vi "Histogram Bin Size Dialog.vi"(8 "error in (no error)":errorcluster, 11 "Current Bin Size":dbl=nan format="%#g") -> (0 "error out":errorcluster, 1 "OK":bool, 2 "Rescale Plot_":bool, 3 "Bin Size_":dbl caption="Bin Size" format="%#g", 5 "Binning Factor_":dbl format="%#g")   [LabVIEW 2021, in "Histogram Window.lvlib"]
doc: "Displays a standard dialog box that prompts users to enter information, such as a user name and password.\n--------------------\n\nThis Express VI is configured as follows:\n\nMessage to Display to the User:Enter new histogram bin size:\nThe inputs are: \nNumber: Bin Size"
uses:
  Histogram Window.lvlib
panel:
  out "Warning":string="< 1 not supported"
  in  "Binning Factor":dbl=1.0 caption="Bin Size" min=1.0 format="%#g"
  in  "Rescale Plot":bool
  out "Current Bin Size":dbl caption="Bin Size" format="%#g"
  in  "New Bin Size":dbl caption="Bin Size" min=0.0 format="%#g"
  out "String":string="Enter new histogram bin size:"
  in  "Cancel":bool
  in  "OK":bool caption="OK2"
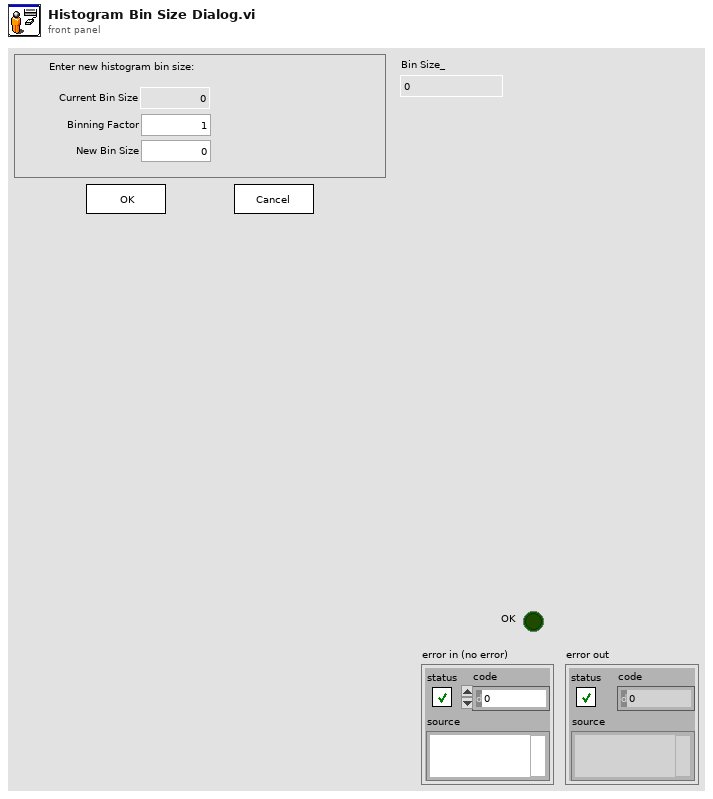
[diagram p1: front panel]
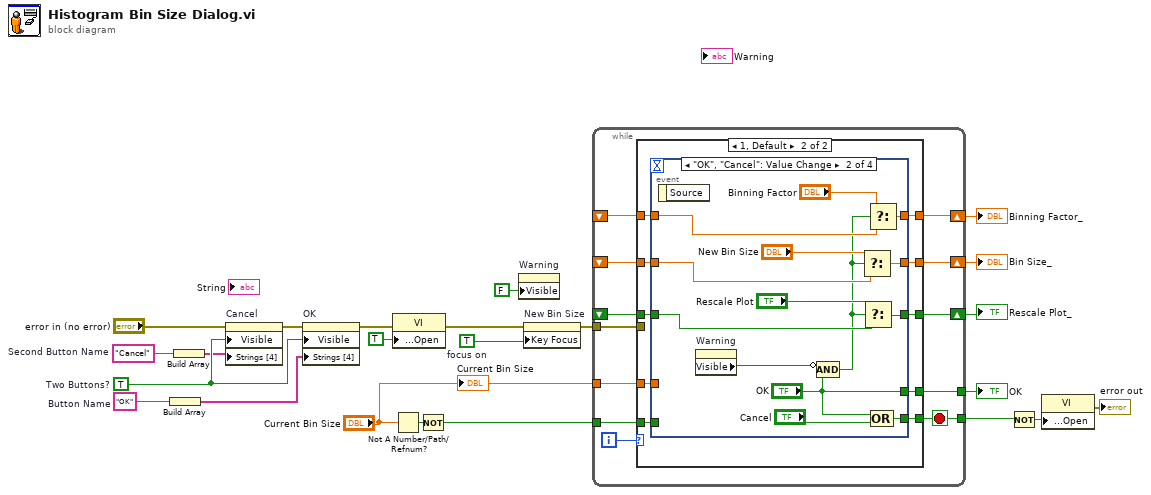
[diagram p0: block diagram]
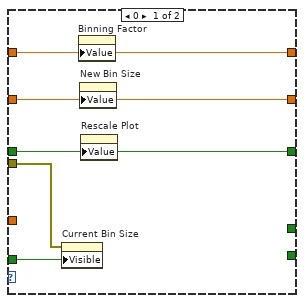
[diagram p2: hidden frame]
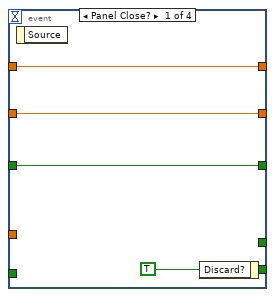
[diagram p3: hidden frame]
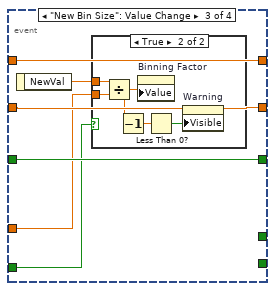
[diagram p4: hidden frame]
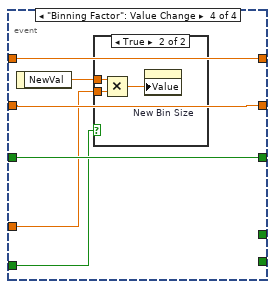
[diagram p6: hidden frame]
diagram:
  w12 = TRUE  # focus on
  w19 = "Cancel"  # Second Button Name
  w17 = "OK"  # Button Name
  w23 = TRUE  # Two Buttons?
  n1 = Build Array(w17) -> (w18:string[])
  n2 = Build Array(w19) -> (w20:string[])
  n3 = property on="Cancel" class="Bool"(error in="error in (no error)", "Visible"=w23, "Strings [4]"=w20) -> (error out=w22:errorcluster)  [unwired: 1 in, 1 out]
  n4 = property on="OK" class="Bool"(error in=w22, "Visible"=w23, "Strings [4]"=w18) -> (error out=w3:errorcluster)  [unwired: 1 in, 1 out]
  n5 = property class="VI"(error in=w3, "Front Panel Window:Open"=TRUE) -> (error out=w16:errorcluster)  [unwired: 1 in, 1 out]
  n6 = Not A Number/Path/Refnum?(number/path/refnum="Current Bin Size") -> (NaN/Path/Refnum?=w2:bool)
  n7 = Not(x=w2) -> (.not. x?=w4:bool)
  n8 = property on="Warning" class="Str"("Visible"=FALSE) -> ()  [unwired: 2 in, 2 out]
  n9 = property on="New Bin Size" class="DigNum (strict)"(error in=w16, "Key Focus"=w12) -> (error out=w5:errorcluster)  [unwired: 1 in, 1 out]
  n10 = while {
    shift-right: [w34] -> w9
    shift-left: _ -> [w33]
    shift-right: [w31] -> w10
    shift-left: _ -> [w32]
    shift-right: [w29] -> w8
    shift-left: _ -> [w30]
    tunnel: [w28] -> w11
    tunnel: [w27] -> w7
    tunnel: "Current Bin Size" -> [w26]
    tunnel: w5 -> [w25]
    tunnel: w4 -> [w24]
    i -> [w35]
    stop <- w27 stop-if-true
    n11 = case shown="1, Default" w35 {
      tunnel: [_ w50] -> w27
      tunnel: [w40 w48] -> w34
      tunnel: w33 -> [w40 w47]
      tunnel: w32 -> [w39 w45]
      tunnel: [w39 w46] -> w31
      tunnel: w30 -> [w38 w43]
      tunnel: [w38 w44] -> w29
      tunnel: [_ w49] -> w28
      tunnel: w26 -> [_ w42]
      tunnel: w25 -> [w37 _]
      tunnel: w24 -> [w36 w41]
      frame 0 {
        n12 = property on="Current Bin Size" class="DigNum (strict)"(error in=w37, "Visible"=w36) -> ()  [unwired: 1 in, 2 out]
        n13 = property on="Binning Factor" class="DigNum (strict)"("Value"=w40) -> ()  [unwired: 2 in, 2 out]
        n14 = property on="New Bin Size" class="DigNum (strict)"("Value"=w39) -> ()  [unwired: 2 in, 2 out]
        n15 = property on="Rescale Plot" class="Bool (strict)"("Value"=w38) -> ()  [unwired: 2 in, 2 out]
      }
      frame 1, Default {
        n16 = event shown="[1] \"OK\", \"Cancel\": Value Change" {
          selector: _ -> [_ _ _ _]
          dyn-events: _ -> [_ _ _ _]
          timeout: _ -> [_ _ _ _]
          tunnel: [w54 w58 _ _] -> w50
          tunnel: [_ "OK" _ _] -> w49
          tunnel: [w53 w67 w74 w85] -> w48
          tunnel: w47 -> [w53 w66 w74 w85]
          tunnel: [w52 w64 w71 w82] -> w46
          tunnel: w45 -> [w52 w63 w71 w82]
          tunnel: [w51 w61 w73 w84] -> w44
          tunnel: w43 -> [w51 w60 w73 w84]
          tunnel: w42 -> [_ _ w70 w81]
          tunnel: w41 -> [_ _ w69 w80]
          event Panel Close? {
            w54 = TRUE ("Discard?")
            n17 = event-data() -> ()  [unwired: 1 in, 1 out]
            n18 = event-data("Discard?"=w54) -> ()  [unwired: 1 in, 1 out]
          }
          event "OK", "Cancel": Value Change {
            n19 = event-data() -> ()  [unwired: 1 in, 1 out]
            n20 = property on="Warning" class="Str"() -> ("Visible"=w57:bool)  [unwired: 2 in, 2 out]
            n21 = Compound Arithmetic op=AND(invert w57, "OK") -> (w55:bool)
            n22 = Select(t="New Bin Size", s=w55, f=w63) -> (s? t:f=w64:dbl)
            n23 = Select(t="Rescale Plot", s=w55, f=w60) -> (s? t:f=w61:bool)
            n24 = Select(t="Binning Factor", s=w55, f=w66) -> (s? t:f=w67:dbl)
            n25 = Compound Arithmetic op=OR("OK", "Cancel") -> (w58:bool)
          }
          event "New Bin Size": Value Change {
            n26 = event-data() -> ("NewVal"=w72:dbl)  [unwired: 1 in]
            n27 = case shown="True" w69 {
              tunnel: w72 -> [_ w79]
              tunnel: w70 -> [_ w78]
              frame False {
              }
              frame True {
                n28 = Divide(x=w79, y=w78) -> (x/y=w77:dbl)
                n29 = Decrement(x=w77) -> (x-1=w76:dbl)
                n30 = property on="Binning Factor" class="DigNum (strict)"("Value"=w77) -> ()  [unwired: 2 in, 2 out]
                n31 = Less Than 0?(x=w76) -> (x < 0?=w75:bool)
                n32 = property on="Warning" class="Str"("Visible"=w75) -> ()  [unwired: 2 in, 2 out]
              }
            }
          }
          event "Binning Factor": Value Change {
            n33 = event-data() -> ("NewVal"=w83:dbl)  [unwired: 1 in]
            n34 = case shown="True" w80 {
              tunnel: w83 -> [_ w88]
              tunnel: w81 -> [_ w86]
              frame False {
              }
              frame True {
                n35 = Multiply(x=w88, y=w86) -> (x*y=w87:dbl)
                n36 = property on="New Bin Size" class="DigNum (strict)"("Value"=w87) -> ()  [unwired: 2 in, 2 out]
              }
            }
          }
        }
      }
    }
  }
  "OK" <- w11
  "Bin Size_" <- w10
  "Rescale Plot_" <- w8
  "Binning Factor_" <- w9
  n37 = Not(x=w7) -> (.not. x?=w21:bool)
  n38 = property class="VI"("Front Panel Window:Open"=w21) -> (error out=→"error out":errorcluster)  [unwired: 2 in, 1 out]
  "Current Bin Size" <- "Current Bin Size"
